vi "Database.vi"(8 "error in (no error)":errorcluster, 9 "Module Routes":refnum<user-event>[](array[refnum]), 11 "Event Registration Refnum":refnum<event-registration>) -> (0 "error out":errorcluster)   [LabVIEW 2016]
doc: "Main for simulated database module."
uses:
  Architecture/Message Queue/Message Cluster.ctl
  Controls/Database Status.ctl
  Car Wash Controller/Controls/Steps.ctl
  Car Wash Controller/Controls/Stations.ctl
  Architecture/Modules.ctl
  Architecture/Message Queue/Message Queue.lvlib
panel:
  in  "debug":bool
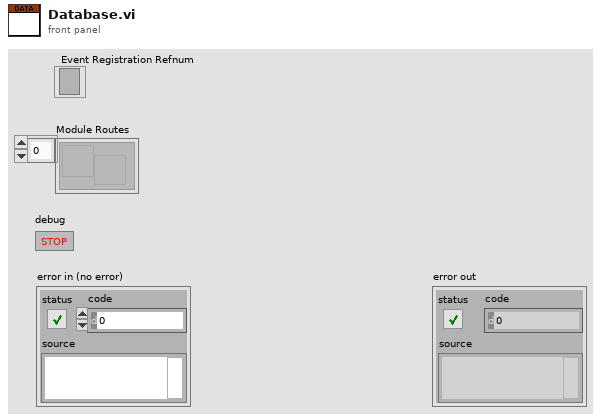
[diagram p1: front panel]
types:
  T1 = typedef "Database Status.ctl" = cluster{"Module Routes":refnum<user-event>[], "Steps":cluster{"Wash Step":T2, "Stations":T3, "Timing (seconds)":u32}[], "Locking Module":T4, "Locked?":bool}
  T2 = typedef "Steps.ctl" = enum16{"Under Body Wash", "Bug Remover", "Pre-Soak", "High Pressure Wash", "Low Pressure Wax", "Spot Free Rinse", "Tire Shine Foam", "Air Dry"}
  T3 = typedef "Stations.ctl" = enum16{"Entry", "Station 1", "Station 2", "Station 3", "Exit"}
  T4 = typedef "Modules.ctl" = enum16{"Database", "Car Wash Controller", "Console"}
  T5 = cluster{"Requested Step":T2, "Requesting Module":T4}
  T6 = cluster{"Requesting Module":T4, "Step Data":cluster{"Wash Step":T2, "Stations":T3, "Timing (seconds)":u32}}
  T7 = typedef "Error Severity.ctl" = enum16{"System Error", "Wash Error", "Minor"}
  T8 = cluster{"Wash Step":T2, "Stations":T3, "Timing (seconds)":u32}
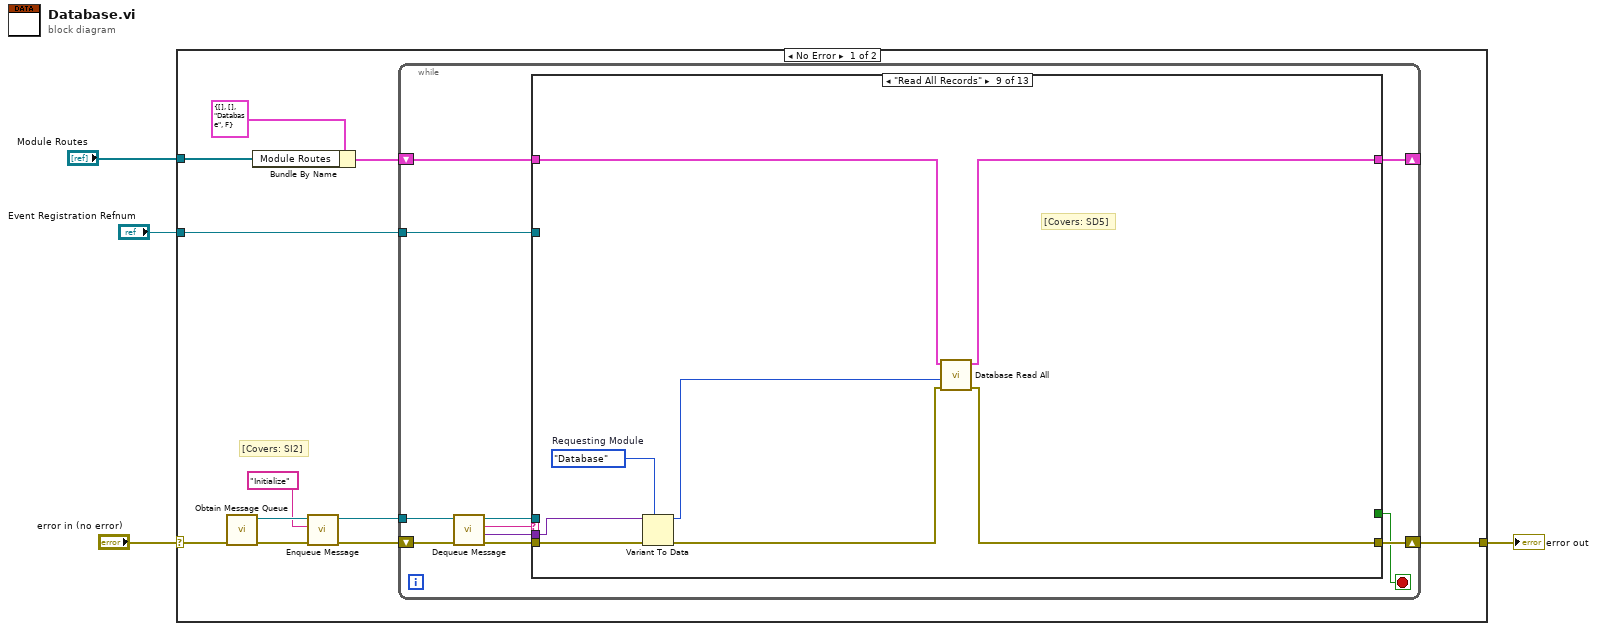
[diagram p0: block diagram]
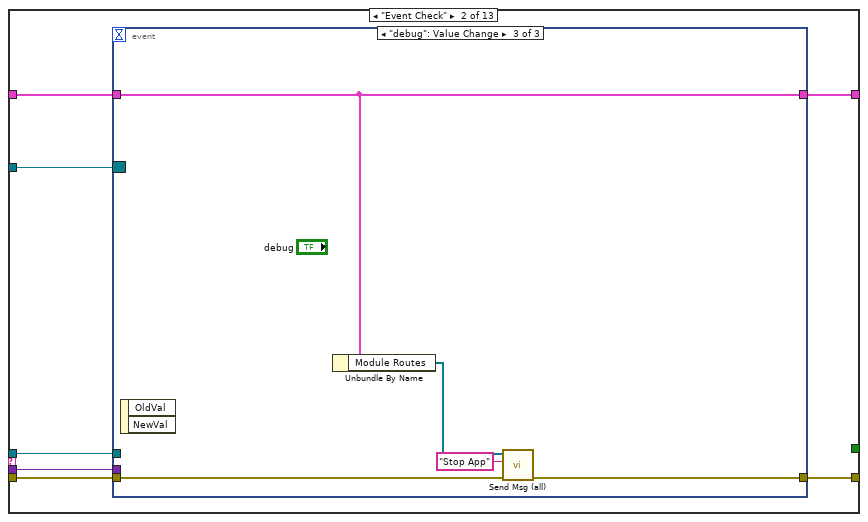
[diagram p3: hidden frame]
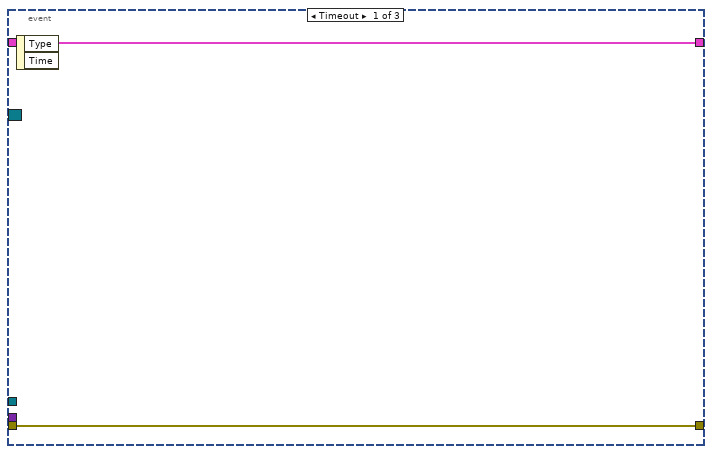
[diagram p4: hidden frame]
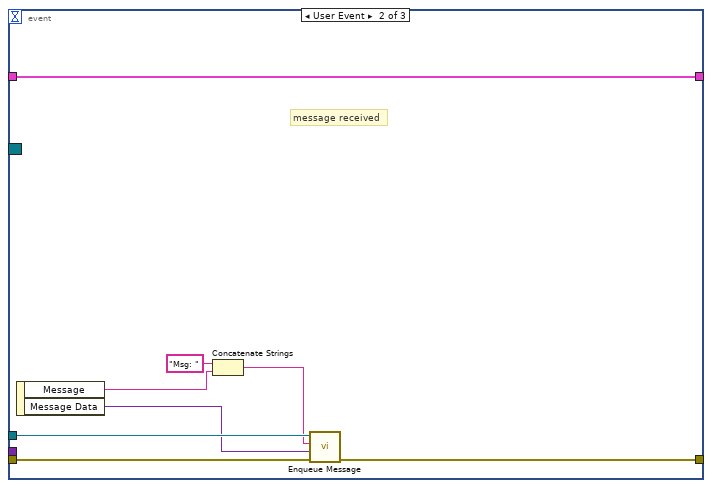
[diagram p5: hidden frame]
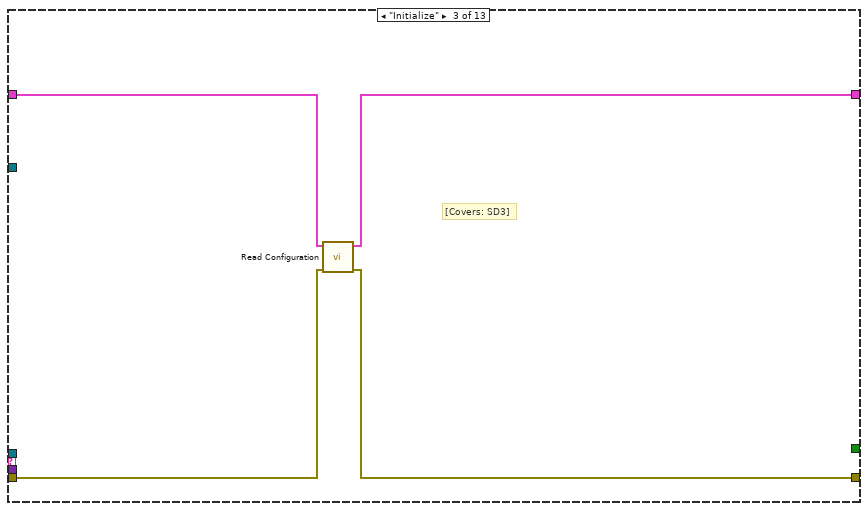
[diagram p6: hidden frame]
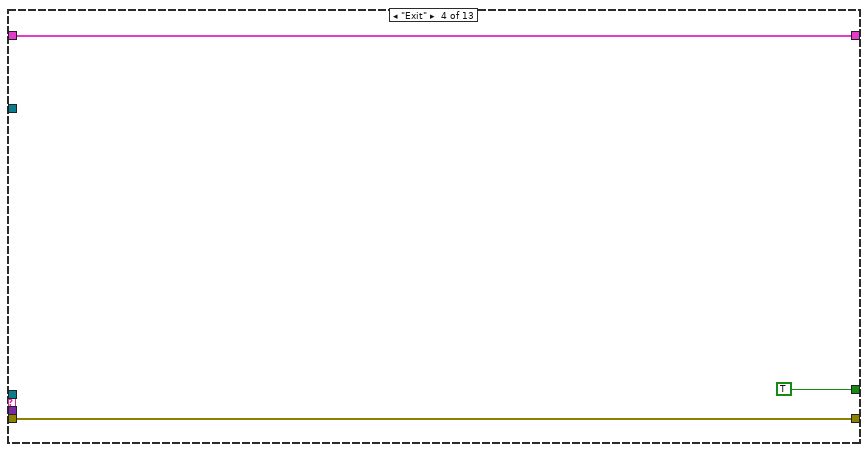
[diagram p7: hidden frame]
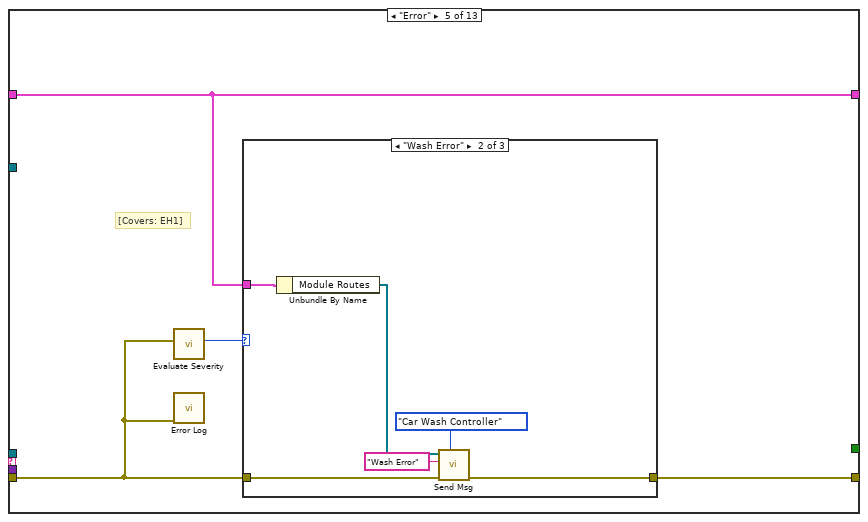
[diagram p8: hidden frame]
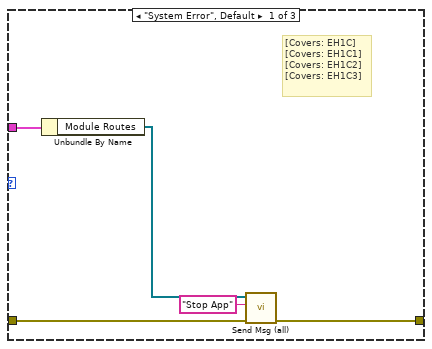
[diagram p9: hidden frame]
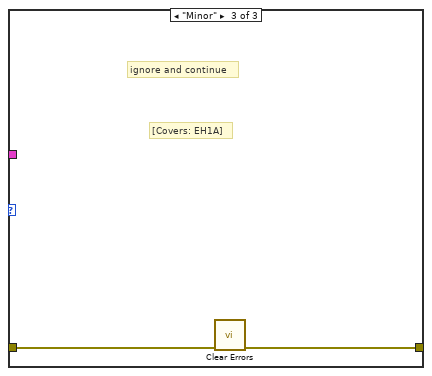
[diagram p10: hidden frame]
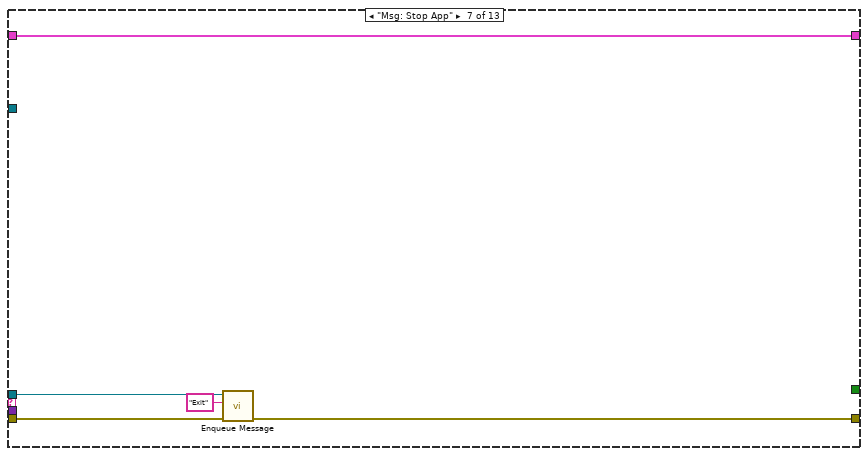
[diagram p12: hidden frame]
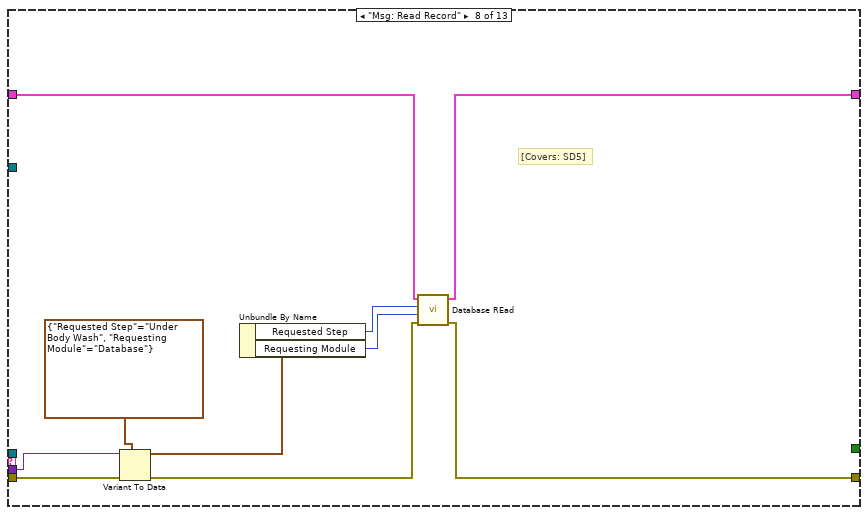
[diagram p13: hidden frame]
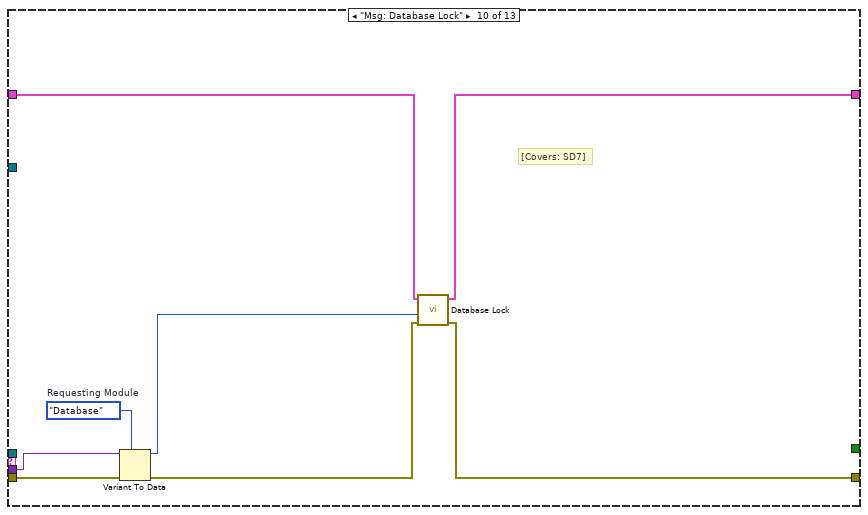
[diagram p14: hidden frame]
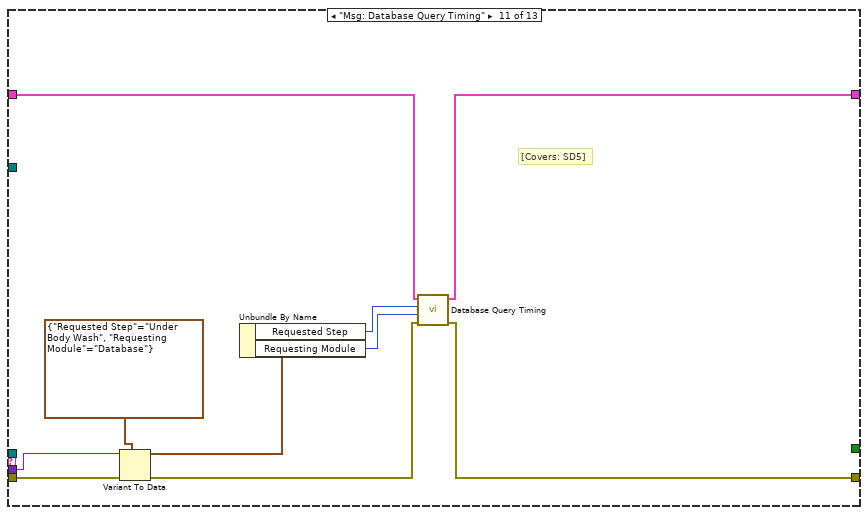
[diagram p15: hidden frame]
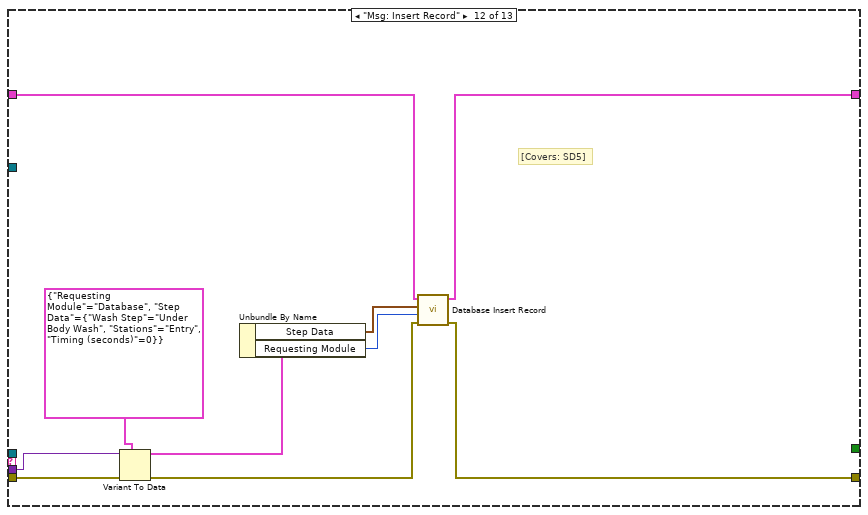
[diagram p16: hidden frame]
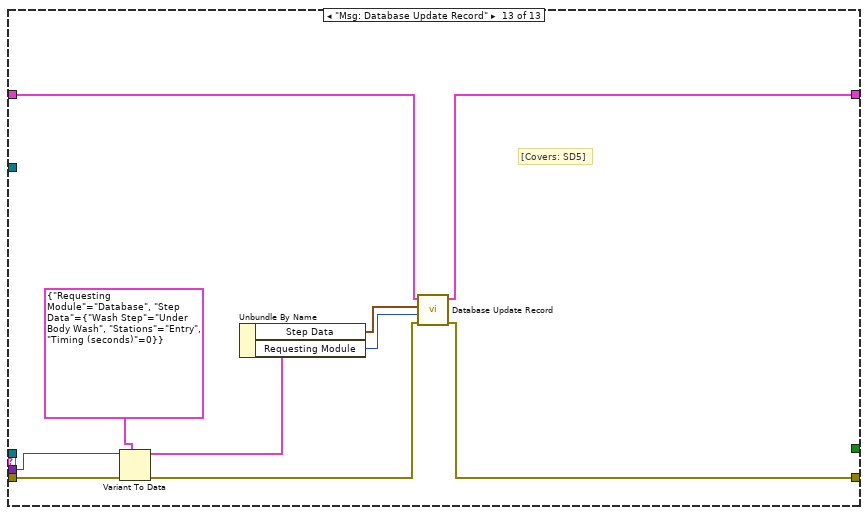
[diagram p17: hidden frame]
diagram:
  n1 = case shown="No Error" "error in (no error)" {
    selector: "error in (no error)" -> [w12 w138]
    tunnel: "Module Routes" -> [w14 _]
    tunnel: "Event Registration Refnum" -> [w13 _]
    tunnel: [w6 w138] -> w1
    frame No Error {
      # "[Covers: SI2]"
      n2 = call "Obtain Message Queue.vi"("error in (no error)"=w12) -> ("error out"=w11:errorcluster, "Message Queue"=w10:refnum<queue>)  [unwired: 9 in]
      n3 = Bundle By Name(cluster=T1 {"Module Routes"=[], "Steps"=[], "Locking Module"=enum."Database", "Locked?"=FALSE} ("Status"), "Module Routes"=w14) -> (w5:T1)
      n4 = call "Enqueue Message.vi"("error in (no error)"=w11, "Message"="Initialize", "Message Queue"=w10) -> ("error out"=w8:errorcluster, "dup Message Queue"=w7:refnum<queue>)  [unwired: 7 in]
      n5 = while {
        tunnel: w13 -> [w26]
        shift-right: [w22] -> w6
        shift-left: w8 -> [w25]
        tunnel: w7 -> [w24]
        shift-right: [w16] -> _
        shift-left: w5 -> [w17]
        stop <- w18 stop-if-true
        n6 = call "Dequeue Message.vi"("error in (no error)"=w25, "Message Queue"=w24) -> ("error out"=w23:errorcluster, "Message Data"=w20:variant, "Message"=w19:string, "dup Message Queue"=w21:refnum<queue>)  [unwired: 6 in]
        n7 = case shown="\"Read All Records\"" w19 {
          tunnel: w26 -> [_ w35 _ _ _ _ _ _ _ _ _ _ _]
          tunnel: w23 -> [w28 w34 w52 w57 w58 w76 w80 w91 w99 w107 w117 w127 w137]
          tunnel: [w28 w33 w51 w57 w60 w76 w78 w86 w94 w102 w112 w122 w132] -> w22
          tunnel: w21 -> [_ w32 _ _ _ _ w79 _ _ _ _ _ _]
          tunnel: w20 -> [_ w31 _ _ _ _ _ w90 w98 w106 w116 w126 w136]
          tunnel: [_ _ _ TRUE _ _ _ _ _ _ _ _ _] -> w18
          tunnel: w17 -> [w27 w30 w54 w55 w59 w75 w81 w88 w96 w104 w114 w124 w134]
          tunnel: [w27 w29 w53 w55 w59 w75 w81 w87 w95 w103 w113 w123 w133] -> w16
          frame Default {
            # "invalid case"
          }
          frame "Event Check" {
            n8 = event shown="[2] \"debug\": Value Change" {
              selector: w35 -> [_ _ _]
              dyn-events: _ -> [_ _ _]
              timeout: _ -> [_ _ _]
              tunnel: [w37 w42 w49] -> w33
              tunnel: w34 -> [w37 w43 w50]
              tunnel: w32 -> [_ w41 _]
              tunnel: w31 -> [_ _ _]
              tunnel: w30 -> [w36 w38 w48]
              tunnel: [w36 w38 w48] -> w29
              event Timeout {
                n9 = event-data() -> ()  [unwired: 1 in, 2 out]
              }
              event User Event {
                # "message received"
                n10 = event-data() -> ("Message"=w44:string, "Message Data"=w40:variant)  [unwired: 1 in]
                n11 = Concatenate Strings("Msg: " ("string"), w44) -> (w39:string)
                n12 = call "Enqueue Message.vi"("error in (no error)"=w43, "Message Data"=w40, "Message"=w39, "Message Queue"=w41) -> ("error out"=w42:errorcluster)  [unwired: 6 in, 1 out]
              }
              event "debug": Value Change {
                n13 = event-data() -> ()  [unwired: 1 in, 2 out]
                n14 = Unbundle By Name(w48) -> ("Module Routes"=w47:refnum<user-event>[])
                n15 = call "Send Msg (all).vi"("error in (no error)"=w50, "Message"="Stop App", "Module Routes"=w47) -> ("error out"=w49:errorcluster)  [unwired: 8 in]
              }
            }
          }
          frame "Initialize" {
            # "[Covers: SD3]"
            n16 = call "Read Configuration.vi"("error in (no error)"=w52, "Status 2"=w54) -> ("error out"=w51:errorcluster, "Status"=w53:T1)  [unwired: 8 in]
          }
          frame "Exit" {
          }
          frame "Error" {
            # "[Covers: EH1]"
            n17 = call "Evaluate Severity.vi"("error in (no error)"=w58) -> ("Severity"=w61:T7)  [unwired: 10 in]
            n18 = call "Error Log.vi"("error in (no error)"=w58) -> ()  [unwired: 11 in]
            n19 = case shown="\"Wash Error\"" w61 {
              tunnel: w58 -> [w66 w72 w74]
              tunnel: [w65 w71 w73] -> w60
              tunnel: w59 -> [w64 w70 _]
              frame "System Error", Default {
                # "[Covers: EH1C]\n[Covers: EH1C1]\n[Covers: EH1C2]\n[Covers: EH1C3]"
                n20 = Unbundle By Name(w64) -> ("Module Routes"=w63:refnum<user-event>[])
                n21 = call "Send Msg (all).vi"("error in (no error)"=w66, "Message"="Stop App", "Module Routes"=w63) -> ("error out"=w65:errorcluster)  [unwired: 8 in]
              }
              frame "Wash Error" {
                n22 = Unbundle By Name(w70) -> ("Module Routes"=w69:refnum<user-event>[])
                n23 = call "Send Msg.vi"("Module"=Modules."Car Wash Controller", "error in (no error)"=w72, "Message"="Wash Error", "Module Routes"=w69) -> ("error out"=w71:errorcluster)  [unwired: 7 in]
              }
              frame "Minor" {
                # "[Covers: EH1A]"
                # "ignore and continue"
                n24 = call <vilib>:"Clear Errors.vi"("error in (no error)"=w74) -> ("error out"=w73:errorcluster)  [unwired: 5 in, 1 out]
              }
            }
          }
          frame "=== Messages ===" {
            # "placeholder"
          }
          frame "Msg: Stop App" {
            n25 = call "Enqueue Message.vi"("error in (no error)"=w80, "Message"="Exit", "Message Queue"=w79) -> ("error out"=w78:errorcluster)  [unwired: 7 in, 1 out]
          }
          frame "Msg: Read Record" {
            # "[Covers: SD5]"
            n26 = Variant To Data(error in=w91, type=T5 {"Requested Step"=enum."Under Body Wash", "Requesting Module"=enum."Database"}, Variant=w90) -> (data=w84:T5, error out=w89:errorcluster)
            n27 = Unbundle By Name(w84) -> ("Requested Step"=w83:T2, "Requesting Module"=w82:T4)
            n28 = call "Database REad.vi"("error in (no error)"=w89, "Requesting Module"=w82, "Requested Step"=w83, "Status"=w88) -> ("error out"=w86:errorcluster, "Status"=w87:T1)  [unwired: 6 in]
          }
          frame "Read All Records" {
            w93 = Modules."Database"  # Requesting Module
            # "[Covers: SD5]"
            n29 = Variant To Data(error in=w99, type=w93, Variant=w98) -> (data=w92:T4, error out=w97:errorcluster)
            n30 = call "Database Read All.vi"("error in (no error)"=w97, "Requesting Module"=w92, "Status"=w96) -> ("error out"=w94:errorcluster, "Status"=w95:T1)  [unwired: 7 in]
          }
          frame "Msg: Database Lock" {
            w101 = Modules."Database"  # Requesting Module
            # "[Covers: SD7]"
            n31 = Variant To Data(error in=w107, type=w101, Variant=w106) -> (data=w100:T4, error out=w105:errorcluster)
            n32 = call "Database Lock.vi"("error in (no error)"=w105, "Requesting Module"=w100, "Status"=w104) -> ("error out"=w102:errorcluster, "Status"=w103:T1)  [unwired: 7 in]
          }
          frame "Msg: Database Query Timing" {
            # "[Covers: SD5]"
            n33 = Variant To Data(error in=w117, type=T5 {"Requested Step"=enum."Under Body Wash", "Requesting Module"=enum."Database"}, Variant=w116) -> (data=w110:T5, error out=w115:errorcluster)
            n34 = Unbundle By Name(w110) -> ("Requested Step"=w109:T2, "Requesting Module"=w108:T4)
            n35 = call "Database Query Timing.vi"("error in (no error)"=w115, "Requesting Module"=w108, "Requested Step"=w109, "Status"=w114) -> ("error out"=w112:errorcluster, "Status"=w113:T1)  [unwired: 6 in]
          }
          frame "Msg: Insert Record" {
            # "[Covers: SD5]"
            n36 = Variant To Data(error in=w127, type=T6 {"Requesting Module"=enum."Database", "Step Data"={"Wash Step"=enum."Under Body Wash", "Stations"=enum."Entry", "Timing (seconds)"=0}}, Variant=w126) -> (data=w120:T6, error out=w125:errorcluster)
            n37 = Unbundle By Name(w120) -> ("Step Data"=w118:T8, "Requesting Module"=w119:T4)
            n38 = call "Database Insert Record.vi"("error in (no error)"=w125, "Requesting Module"=w119, "Step Data"=w118, "Status"=w124) -> ("error out"=w122:errorcluster, "Status"=w123:T1)  [unwired: 6 in]
          }
          frame "Msg: Database Update Record" {
            # "[Covers: SD5]"
            n39 = Variant To Data(error in=w137, type=T6 {"Requesting Module"=enum."Database", "Step Data"={"Wash Step"=enum."Under Body Wash", "Stations"=enum."Entry", "Timing (seconds)"=0}}, Variant=w136) -> (data=w130:T6, error out=w135:errorcluster)
            n40 = Unbundle By Name(w130) -> ("Step Data"=w128:T8, "Requesting Module"=w129:T4)
            n41 = call "Database Update Record.vi"("error in (no error)"=w135, "Requesting Module"=w129, "Step Data"=w128, "Status"=w134) -> ("error out"=w132:errorcluster, "Status"=w133:T1)  [unwired: 6 in]
          }
        }
      }
    }
    frame Error {
    }
  }
  "error out" <- w1
